vi "Pre Launch Init.vi"(11 "GUI in":refnum<class "GUI.lvclass">) -> (0 "error out":errorcluster, 3 "GUI out":refnum<class "GUI.lvclass">)   [LabVIEW 2020, in "GUI.lvlib" / "GUI.lvclass"]
doc: "Initializes the panel actor. Creates the Panel Helper.\n\n----\nPlease see the following web address for additional documentation and tutorial information:\nhttp://www.mooregoodideas.com/mgi-panel-manager/\n\nAuthor: Derek Trepanier\n\nCopyright (c) 2018, Moore Good Ideas, Inc.\n\nAll rights reserved.\n\nRedistribution and use in source and binary forms, with or without modification, are permitted provided that the following conditions are met:\n\n * Redistributions of source code must retain the above copyright notice, this list of conditions and the following disclaimer.\n * Redistributions in binary form must reproduce the above copyright notice, this list of conditions and the following disclaimer in the documentation and/or other materials provided with the distribution.\n * Neither the name of Moore Good Ideas, Inc. nor the names of its contributors may be used to endorse or promote products derived from this software without specific prior written permission.\n\nTHIS SOFTWARE IS PROVIDED BY THE COPYRIGHT HOLDERS AND CONTRIBUTORS \"AS IS\" AND ANY EXPRESS OR IMPLIED WARRANTIES, INCLUDING, BUT NOT LIMITED TO, THE IMPLIED WARRANTIES OF MERCHANTABILITY AND FITNESS FOR A PARTICULAR PURPOSE ARE DISCLAIMED. IN NO EVENT SHALL THE COPYRIGHT OWNER OR CONTRIBUTORS BE LIABLE FOR ANY DIRECT, INDIRECT, INCIDENTAL, SPECIAL, EXEMPLARY, OR CONSEQUENTIAL DAMAGES (INCLUDING, BUT NOT LIMITED TO, PROCUREMENT OF SUBSTITUTE GOODS OR SERVICES; LOSS OF USE, DATA, OR PROFITS; OR BUSINESS INTERRUPTION) HOWEVER CAUSED AND ON ANY THEORY OF LIABILITY, WHETHER IN CONTRACT, STRICT LIABILITY, OR TORT (INCLUDING NEGLIGENCE OR OTHERWISE) ARISING IN ANY WAY OUT OF THE USE OF THIS SOFTWARE, EVEN IF ADVISED OF THE POSSIBILITY OF SUCH DAMAGE."
uses:
  GUI.lvclass
  <vilib>/ActorFramework/Message Enqueuer/Message Enqueuer.lvclass
  Task info df.ctl
  Collection State df.ctl
  Task selection df.ctl
  Automate df.ctl
  GUI.lvclass/GUI.ctl
  <vilib>/MGI/Panel Manager/Panel Actor/Panel Actor/Panel Actor.lvclass
  <vilib>/Utility/config.llb/NI_LVConfig.lvlib
panel:
  in  "Config Array":string[][](array[string])
  in  "Path":path
  in  "Force Task Enq":refnum<class "Message Enqueuer.lvclass">
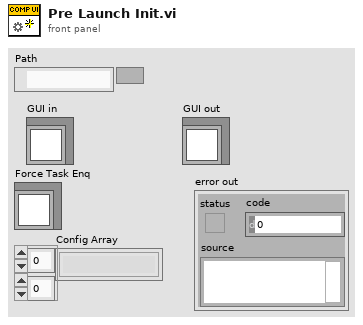
[diagram p1: front panel]
types:
  T1 = typedef "Automate df.ctl" = cluster{"Automate?":bool, "Num Parabs":u16, "Patterns Array":u8[][], "Phase Array":i32[][]}
  T2 = typedef "Task selection df.ctl" = cluster{"Task Type Select":enum32{"Frequency Task", "Scanning Task"}, "Input Select Type":enum32{"Force Input", "Movement Input"}, "Collect EMG?":bool, "Collect acceleration?":bool, "EMG Rate":u16, "Acceleration Rate":u16}
  T3 = typedef "Collection State df.ctl" = enum16{"Start", "Collection", "Stop", "Trial Pause", "Break Collection"}
  T4 = typedef "Task info df.ctl" = cluster{"Number of Trials":u8, "Sampling Rate (Hz)":u16, "Trial Duration (s)":u8, "Adjusted MVC (N)":dbl, "R Phase":i32, "L Phase":i32, "L Pattern":u8, "R Pattern":u8, "Time Between Trials (s)":u8, "Lissajous Speed":u16}
  T5 = typedef "NI_LVConfig.lvlib/Config Data RefNum.ctl" = refnum<k1>
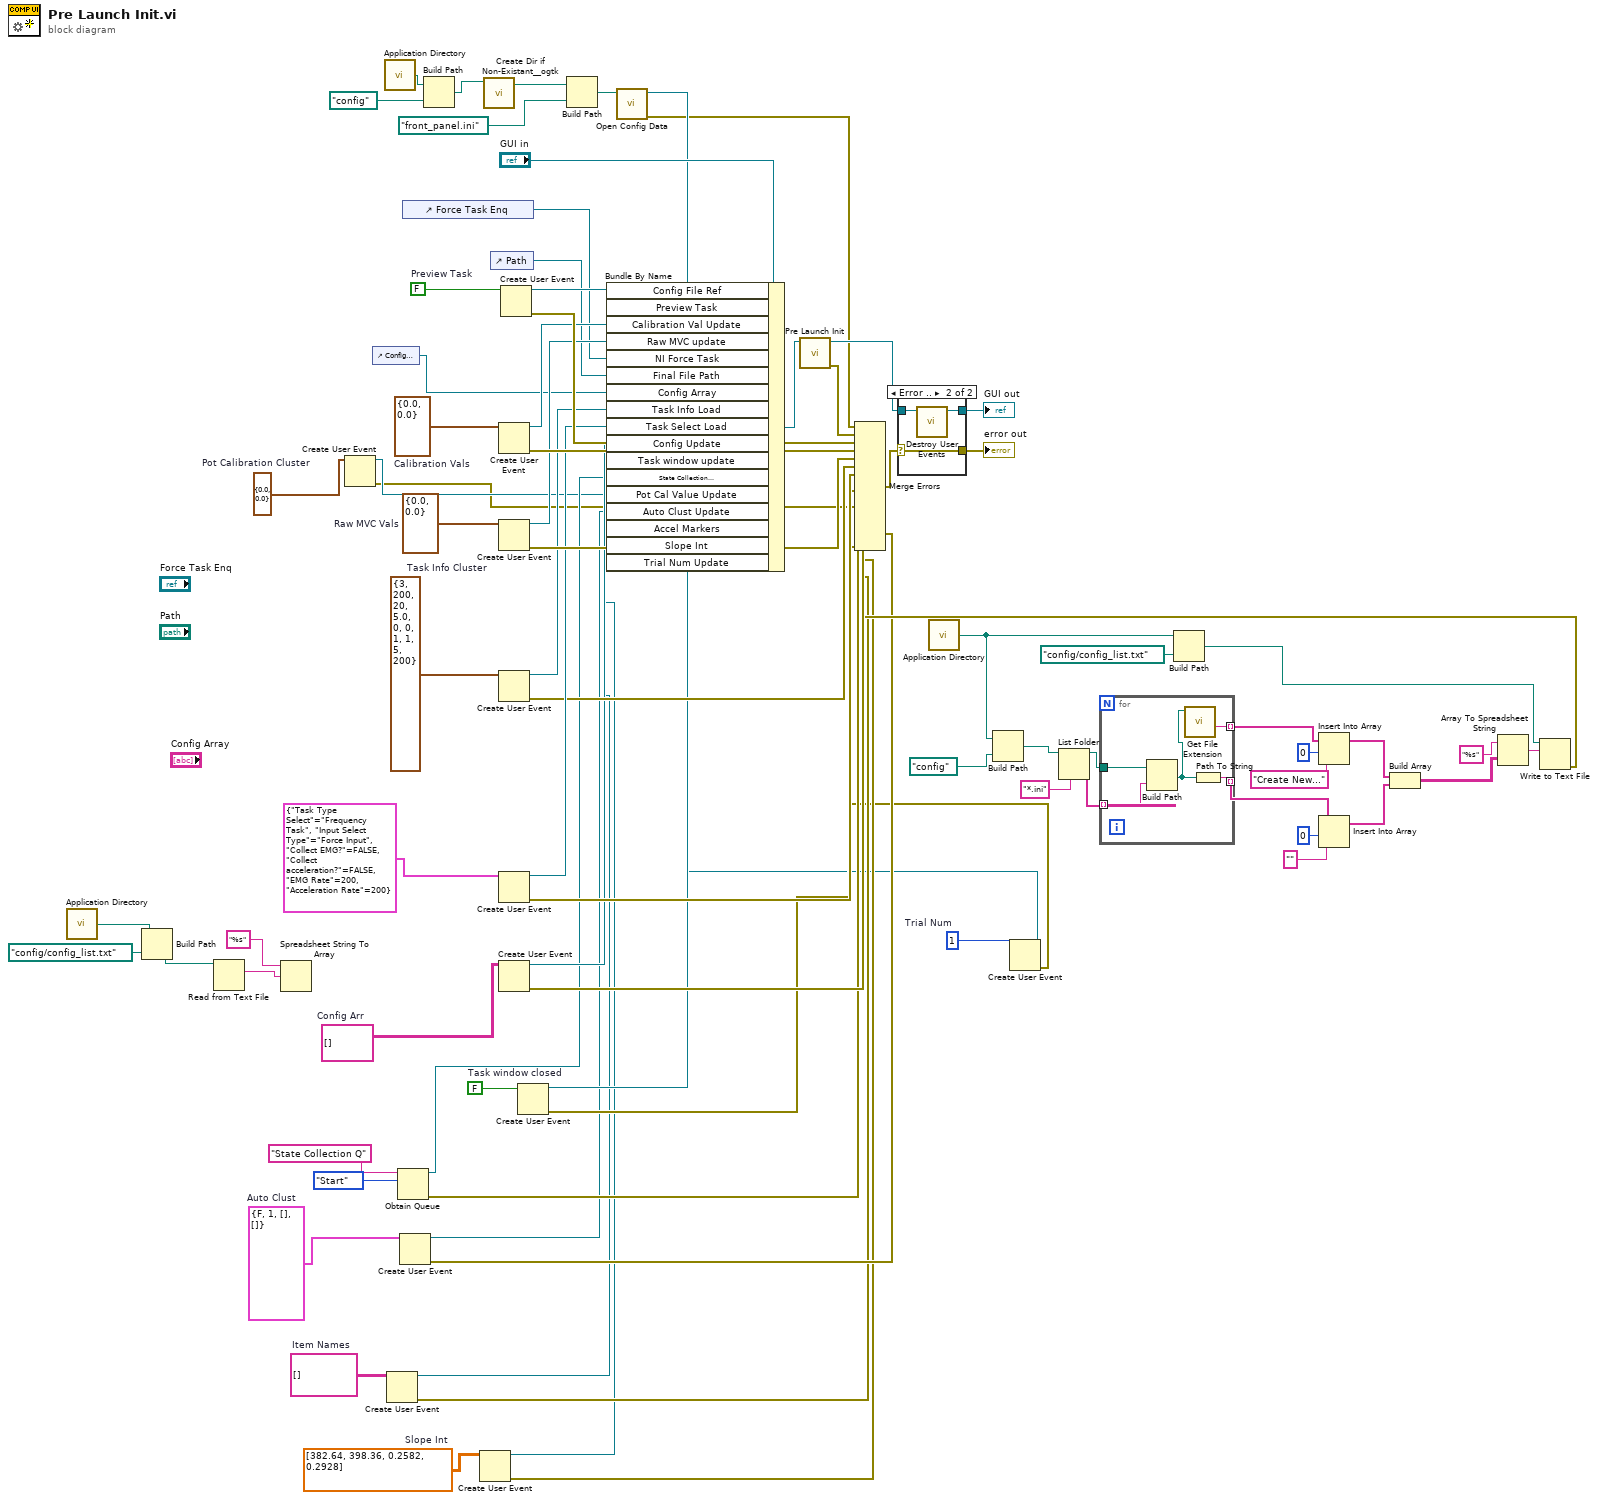
[diagram p0: block diagram]
diagram:
  w3 = 1  # Trial Num
  w6 = dbl[][] [[382.64, 398.36], [0.2582, 0.2928]]  # Slope Int
  w9 = string[][] []  # Item Names
  w12 = T1 {"Automate?"=FALSE, "Num Parabs"=1, "Patterns Array"=[], "Phase Array"=[]}  # Auto Clust
  w36 = cluster{"Left 2":dbl, "Right 2":dbl} {"Left 2"=0.0, "Right 2"=0.0}  # Pot Calibration Cluster
  w43 = FALSE  # Task window closed
  w44 = string[][] []  # Config Arr
  w63 = T4 {"Number of Trials"=3, "Sampling Rate (Hz)"=200, "Trial Duration (s)"=20, "Adjusted MVC (N)"=5.0, "R Phase"=0, "L Phase"=0, "L Pattern"=1, "R Pattern"=1, "Time Between Trials (s)"=5, "Lissajous Speed"=200}  # Task Info Cluster
  w70 = cluster{"Left":dbl, "Right":dbl} {"Left"=0.0, "Right"=0.0}  # Raw MVC Vals
  w73 = cluster{"Left":dbl, "Right":dbl} {"Left"=0.0, "Right"=0.0}  # Calibration Vals
  w83 = FALSE  # Preview Task
  n1 = call <vilib>:"Application Directory.vi"() -> ("Application Directory"=w49:path)
  n2 = Build Path(base path=w49, name or relative path=path "config/config_list.txt") -> (appended path=w47:path)
  n3 = Read from Text File(file (use dialog)=w47) -> (text=w46:string)  [unwired: 3 in, 3 out]
  n4 = Spreadsheet String To Array(format string="%s", spreadsheet string=w46) -> ()  [unwired: 2 in, 1 out]
  n5 = Create User Event(user event datatype=w36) -> (user event=w35:refnum<user-event>, error out=w34:errorcluster)  [unwired: 1 in]
  n6 = control-ref of="Config Array"() -> (w50:refnum<vi>)
  n7 = call <vilib>:"Application Directory.vi"() -> ("Application Directory"=w64:path)
  n8 = Create User Event(user event datatype=w9) -> (user event=w8:refnum<user-event>, error out=w7:errorcluster)  [unwired: 1 in]
  n9 = Obtain Queue(name (unnamed)="State Collection Q", element data type=Collection_State_df."Start" ("Collection State")) -> (queue out=w38:refnum<queue>, error out=w37:errorcluster)  [unwired: 3 in, 1 out]
  n10 = Create User Event(user event datatype=w12) -> (user event=w10:refnum<user-event>, error out=w11:errorcluster)  [unwired: 1 in]
  n11 = control-ref of="Force Task Enq"() -> (w67:refnum<vi>)
  n12 = Build Path(base path=w64, name or relative path=path "config") -> (appended path=w58:path)
  n13 = Create User Event(user event datatype=w6) -> (user event=w4:refnum<user-event>, error out=w5:errorcluster)  [unwired: 1 in]
  n14 = call <userlib>:"Create Dir if Non-Existant__ogtk.vi"("Directory Path"=w58) -> ("dup Directory Path"=w56:path)  [unwired: 8 in, 2 out]
  n15 = control-ref of="Path"() -> (w65:refnum<vi>)
  n16 = Create User Event(user event datatype=w73) -> (user event=w72:refnum<user-event>, error out=w71:errorcluster)  [unwired: 1 in]
  n17 = Create User Event(user event datatype=w70) -> (user event=w69:refnum<user-event>, error out=w68:errorcluster)  [unwired: 1 in]
  n18 = Create User Event(user event datatype=w63) -> (user event=w62:refnum<user-event>, error out=w60:errorcluster)  [unwired: 1 in]
  n19 = Create User Event(user event datatype=T2 {"Task Type Select"=enum."Frequency Task", "Input Select Type"=enum."Force Input", "Collect EMG?"=FALSE, "Collect acceleration?"=FALSE, "EMG Rate"=200, "Acceleration Rate"=200} ("Task Selection")) -> (user event=w61:refnum<user-event>, error out=w59:errorcluster)  [unwired: 1 in]
  n20 = Create User Event(user event datatype=w44) -> (user event=w52:refnum<user-event>, error out=w51:errorcluster)  [unwired: 1 in]
  n21 = Create User Event(user event datatype=w83) -> (user event=w80:refnum<user-event>, error out=w78:errorcluster)  [unwired: 1 in]
  n22 = Create User Event(user event datatype=w43) -> (user event=w42:refnum<user-event>, error out=w41:errorcluster)  [unwired: 1 in]
  n23 = Build Path(base path=w56, name or relative path=path "front_panel.ini") -> (appended path=w55:path)
  n24 = call <vilib>:"Open Config Data.vi"("configuration file path"=w55) -> ("error out"=w53:errorcluster, "refnum"=w54:T5)  [unwired: 8 in, 1 out]
  n25 = call <vilib>:"Application Directory.vi"() -> ("Application Directory"=w26:path)
  n26 = Build Path(base path=w26, name or relative path=path "config") -> (appended path=w31:path)
  n27 = Create User Event(user event datatype=w3) -> (user event=w1:refnum<user-event>, error out=w2:errorcluster)  [unwired: 1 in]
  n28 = Bundle By Name(cluster="GUI in", "Config File Ref"=w54, "Preview Task"=w80, "Calibration Val Update"=w72, "Raw MVC update"=w69, "NI Force Task"=w67, "Final File Path"=w65, "Config Array"=w50, "Task Info Load"=w62, "Task Select Load"=w61, "Config Update"=w52, "Task window update"=w42, "State Collection \nQ"=w38, "Pot Cal Value Update"=w35, "Auto Clust Update"=w10, "Accel Markers"=w8, "Slope Int"=w4, "Trial Num Update"=w1) -> (w81:refnum<class "GUI.lvclass">)
  n29 = call-parent "Pre Launch Init.vi"("Panel Actor in"=w81) -> ("error out"=w79:errorcluster, "Panel Actor out"=w77:refnum<class "GUI.lvclass">)  [unwired: 9 in]
  n30 = List Folder(path=w31, pattern="*.ini") -> (path out=w15:path, filenames=w24:string[])  [unwired: 2 in, 2 out]
  n31 = for {
    tunnel: w24 -> [w88] mode=indexing
    tunnel: w15 -> [w86]
    tunnel: [w87] -> w25 mode=indexing
    tunnel: [w85] -> w14 mode=indexing
    n32 = Build Path(base path=w86, name or relative path=w88) -> (appended path=w84:path)
    n33 = call <vilib>:"Get File Extension.vi"("file"=w84) -> ("filename without extension"=w85:string)  [unwired: 6 in, 4 out]
    n34 = Path To String(path=w84) -> (string=w87:string)
  }
  n35 = Build Path(base path=w26, name or relative path=path "config/config_list.txt") -> (appended path=w29:path)
  n36 = Insert Into Array(array=w14, index=0, new element="Create New..." ("new element/subarray")) -> (w19:string[])
  n37 = Insert Into Array(array=w25, index=0, new element="" ("new element/subarray")) -> (w18:string[])
  n38 = Build Array(w19, w18) -> (w17:string[][])
  n39 = Array To Spreadsheet String(array=w17, 3:"%s" ("format string")) -> (spreadsheet string=w27:string)  [unwired: 1 in]
  n40 = Write to Text File(file (use dialog)=w29, text=w27) -> (error out=w16:errorcluster)  [unwired: 2 in, 2 out]
  n41 = Merge Errors(w53, w79, w78, w71, w68, w60, w59, w51, w41, w37, w34, w16, w11, w7, w5, w2) -> (w75:errorcluster)
  n42 = case shown="Error .." w75 {
    selector: w75 -> [w89 w91]
    tunnel: [w90 w92] -> w76
    tunnel: w77 -> [w90 w93]
    tunnel: [w89 w91] -> w74
    frame No Error {
    }
    frame Error {
      n43 = call "Destroy User Events.vi"("GUI in"=w93) -> ("GUI out"=w92:refnum<class "GUI.lvclass">)  [unwired: 9 in, 1 out]
    }
  }
  "error out" <- w74
  "GUI out" <- w76
